vi "有协议模式.vi"(8 "错误输入（无错误）":errorcluster, 9 "等待时间":u32, 10 "写入命令":string, 11 "VISA资源名称":refnum<visa-resource-name>) -> (0 "错误输出":errorcluster, 2 "通讯数据":string, 3 "VISA资源名称输出":refnum<visa-resource-name>)   [LabVIEW 2017]
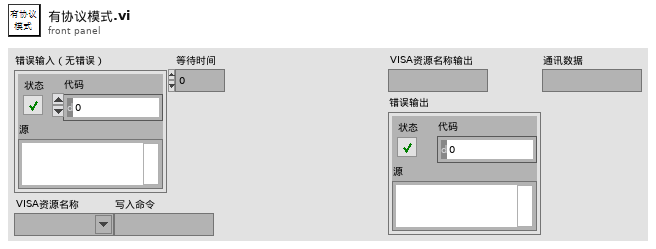
[diagram p1: front panel]
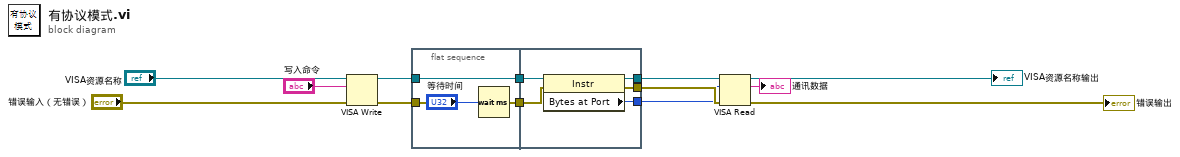
[diagram p0: block diagram]
diagram:
  n1 = VISA Write(VISA resource name="VISA资源名称", write buffer="写入命令", error in (no error)="错误输入（无错误）") -> (VISA resource name out=w9:refnum<visa-resource-name>, error out=w7:errorcluster)  [unwired: 1 out]
  n2 = flat-sequence {
    tunnel: [w15] -> w10
    tunnel: w9 -> [w15]
    tunnel: [w14] -> w8
    tunnel: w7 -> [w14]
    tunnel: w10 -> [w21]
    tunnel: w8 -> [w20]
    tunnel: [w19] -> w6
    tunnel: [w18] -> w5
    tunnel: [w17] -> w4
    frame #0 {
      n3 = Wait (ms)(milliseconds to wait="等待时间") -> ()  [unwired: 1 out]
    }
    frame #1 {
      n4 = property class="Instr"(reference=w21, error in=w20) -> (reference out=w19:refnum<visa-resource-name>, error out=w18:errorcluster, "Bytes at Port"=w17:u32)
    }
  }
  n5 = VISA Read(VISA resource name=w6, byte count=w4, error in (no error)=w5) -> (VISA resource name out=→"VISA资源名称输出":refnum<visa-resource-name>, read buffer=→"通讯数据":string, error out=→"错误输出":errorcluster)  [unwired: 1 out]
